vi "Progress.vi"(8 "error in (no error)":errorcluster, 9 "Sweep % Complete (0-1)":dbl, 11 "ExecutionStatus in":refnum<class "ExecutionStatus.lvclass">) -> (0 "error out":errorcluster, 1 "% Complete (0-100)":dbl, 3 "ExecutionStatus out":refnum<class "ExecutionStatus.lvclass">)   [LabVIEW 2019, in "ExecutionStatus.lvclass"]
uses:
  ExecutionStatus.lvclass
  ExecutionStatus.lvclass/ExecutionStatus.ctl
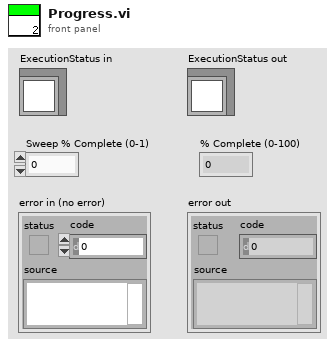
[diagram p1: front panel]
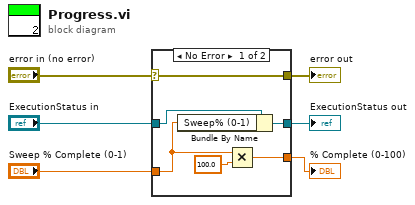
[diagram p0: block diagram]
diagram:
  n1 = case shown="No Error" "error in (no error)" {
    selector: "error in (no error)" -> [w12 w14]
    tunnel: [w12 w14] -> w5
    tunnel: [w10 w13] -> w3
    tunnel: "ExecutionStatus in" -> [w11 w13]
    tunnel: "Sweep % Complete (0-1)" -> [w7 _]
    tunnel: [w8 _] -> w1
    frame No Error {
      n2 = Bundle By Name(cluster=w11, "Sweep% (0-1)"=w7) -> (w10:refnum<class "ExecutionStatus.lvclass">)
      n3 = Multiply(x=w7, y=100.0) -> (x*y=w8:dbl)
    }
    frame Error {
    }
  }
  "error out" <- w5
  "ExecutionStatus out" <- w3
  "% Complete (0-100)" <- w1
